vi "SSMObtainRequestEvents.vi"(8 "error in (no error)":errorcluster, 10 "CreateNew (F)":bool) -> (0 "error out":errorcluster, 2 "SSMRequestEvents":T1)   [LabVIEW 2018, in "Test.lvclass"]
uses:
  Test.lvclass
  SSMRequestEvents.ctl
  SSMEventType.ctl
panel:
  # "If you want to add other Request Events, open this typedef, copy an existing event and rename it to your Request name.\n\nNext create a typedef for the  data and put it into PublicAPI/Arguments/Requests\n\nNext, add an event handler loop event case in Main.vi to handle the new request event\n\nMost likely, each request will also require the creation of a new Queued Message Handler loop case in Main.VI"
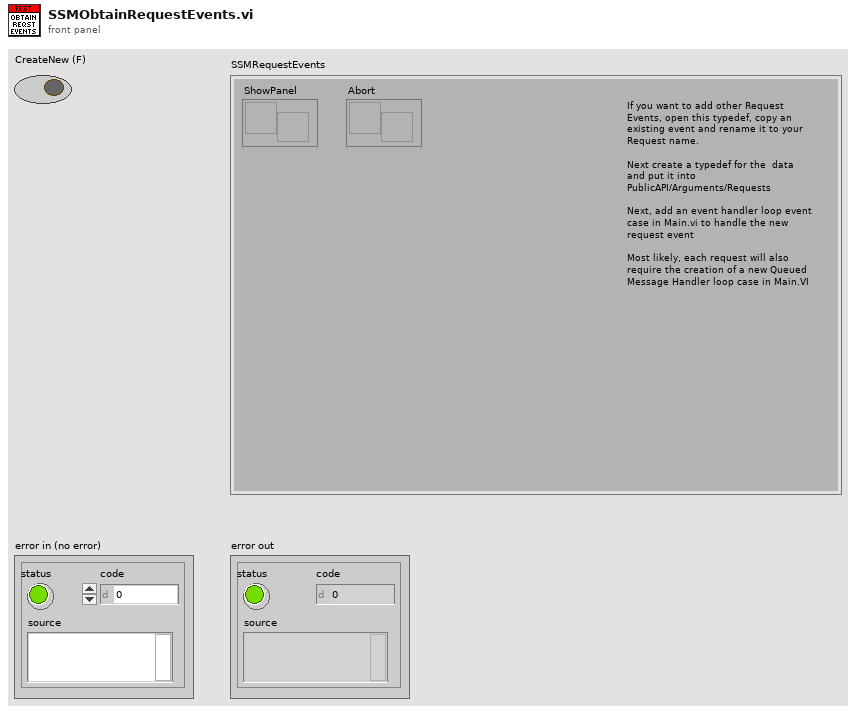
[diagram p1: front panel]
types:
  T1 = typedef "Test.lvclass/SSMRequestEvents.ctl" = cluster{"ShowPanel":refnum<user-event>, "Abort":refnum<user-event>}
  T2 = typedef "Test.lvclass/SSMEventType.ctl" = cluster{"Requester":string, "Data":variant}
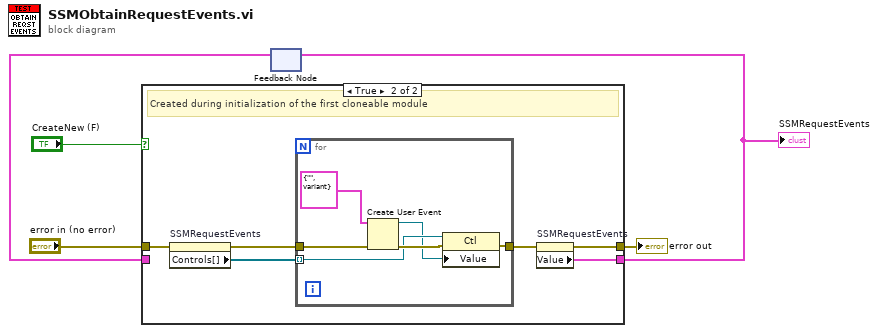
[diagram p0: block diagram]
diagram:
  n1 = feedback #1() -> (w3:T1)  [unwired: 1 in]
  n2 = case shown="True" "CreateNew (F)" {
    tunnel: "error in (no error)" -> [w7 w13]
    tunnel: w3 -> [w6 _]
    tunnel: [w7 w9] -> w2
    tunnel: [w6 w8] -> w1
    frame False {
    }
    frame True {
      # "Created during initialization of the first cloneable module"
      n3 = property on="SSMRequestEvents" class="Clust (strict)"(error in=w13) -> (error out=w12:errorcluster, "Controls[]"=w11:refnum<vi>[])  [unwired: 1 in, 1 out]
      n4 = for {
        tunnel: w11 -> [w15] mode=indexing
        tunnel: w12 -> [w18]
        tunnel: [w16] -> w10
        n5 = Create User Event(user event datatype=T2 {"Requester"="", "Data"=variant} ("clEventType"), error in=w18) -> (user event=w14:refnum<user-event>, error out=w17:errorcluster)
        n6 = property on="Property Node" class="Ctl"(reference=w15, error in=w17, "Value"=w14) -> (error out=w16:errorcluster)  [unwired: 1 out]
      }
      n7 = property on="SSMRequestEvents" class="Clust (strict)"(error in=w10) -> (error out=w9:errorcluster, "Value"=w8:T1)  [unwired: 1 in, 1 out]
    }
  }
  "error out" <- w2
  "SSMRequestEvents" <- w1
  n8 = feedback-in #1(w1) -> ()
